vi "MessageBase.getParameters.vi"(8 "error in":errorcluster, 10 "Variant":variant, 11 "MessageBase in":refnum<class "MessageBase.lvclass">) -> (0 "error out":errorcluster, 2 "Variant":variant, 3 "MessageBase out":refnum<class "MessageBase.lvclass">)   [LabVIEW 2020, in "MessageBase.lvclass"]
uses:
  MessageBase.lvclass
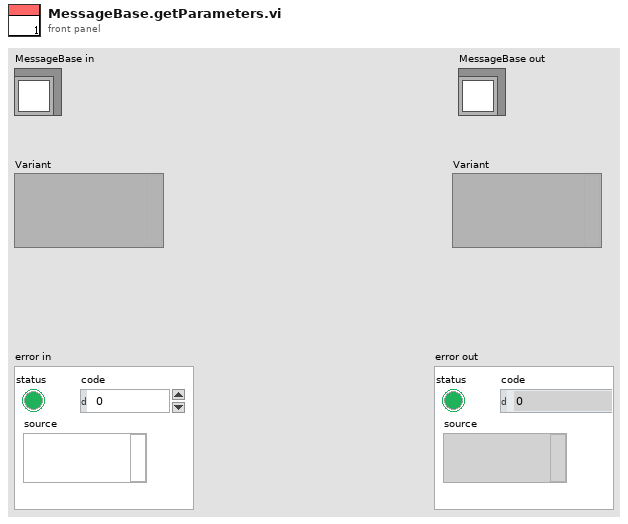
[diagram p1: front panel]
types:
  T1 = typedef "FieldSpec.ctl" = cluster{"Name":string, "Offset":i32, "Length":i32, "FieldType":enum16{"Alphanumeric", "Binary", "BinaryLongPrice", "BinaryShortPrice", "BitField", "PrintableAscii", "Value"}, "FieldValue":variant}
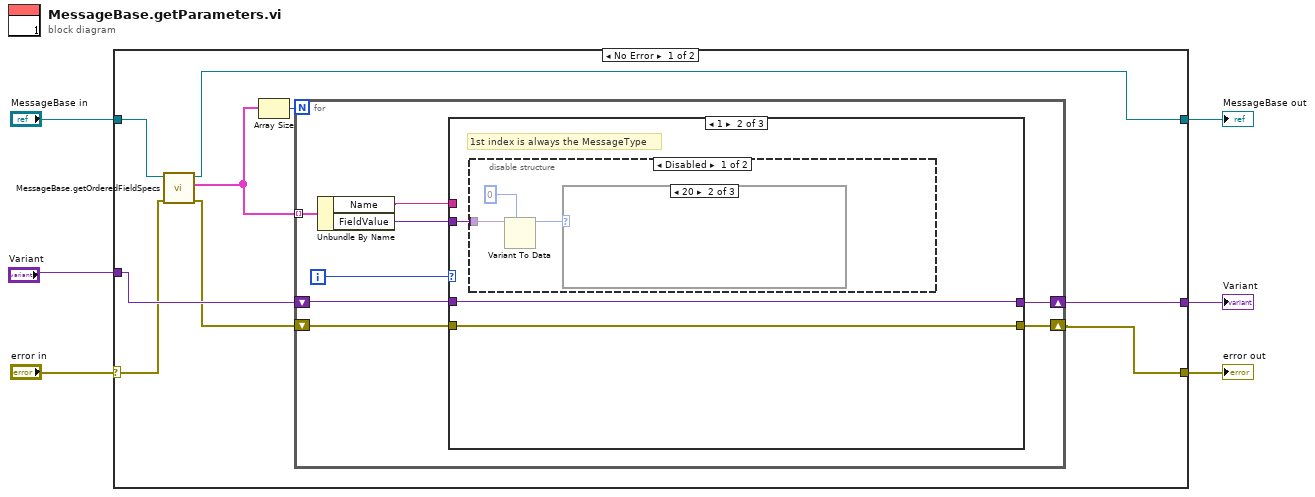
[diagram p0: block diagram]
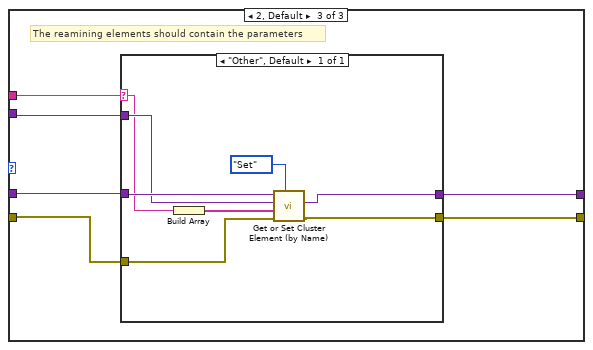
[diagram p6: hidden frame]
diagram:
  n1 = case shown="No Error" "error in" {
    selector: "error in" -> [w10 w47]
    tunnel: [w8 w47] -> w5
    tunnel: [w9 w46] -> w3
    tunnel: "MessageBase in" -> [w14 w46]
    tunnel: "Variant" -> [w12 _]
    tunnel: [w11 _] -> w1
    frame No Error {
      n2 = call-dynamic "MessageBase.getOrderedFieldSpecs.vi"("error in (no error)"=w10, "MessageBase in"=w14) -> ("error out"=w7:errorcluster, "OrderedFieldSpecs"=w13:T1[], "MessageBase out"=w9:refnum<class "MessageBase.lvclass">)  [unwired: 7 in]
      n3 = Array Size(array=w13) -> (size(s)=w15:i32)
      n4 = for {
        N: w15 -> [_]
        tunnel: w13 -> [w23] mode=indexing
        shift-right: [w19] -> w11
        shift-left: w12 -> [w18]
        shift-right: [w17] -> w8
        shift-left: w7 -> [w16]
        i -> [w22]
        n5 = Unbundle By Name(w23) -> ("Name"=w20:string, "FieldValue"=w21:variant)
        n6 = case shown="1" w22 {
          tunnel: w21 -> [_ w28 w36]
          tunnel: w20 -> [_ _ w37]
          tunnel: [w25 w27 w35] -> w19
          tunnel: w18 -> [w25 w27 w34]
          tunnel: [w24 w26 w33] -> w17
          tunnel: w16 -> [w24 w26 w32]
          frame 0 {
            # "0th element is the Message Length"
          }
          frame 1 {
            # "1st index is always the MessageType"
            n7 = disable-structure shown="Disabled" {
              disable-tunnel: w28 -> [w30 _]
              frame Disabled {
                n8 = Variant To Data(type=u8 0, Variant=w30) -> (data=w29:u8)  [unwired: 1 in, 1 out]
                n9 = case shown="20" w29 {
                  frame 0, Default {
                  }
                  frame 32 {
                  }
                  frame 33 {
                  }
                }
              }
              frame Enabled {
              }
            }
          }
          frame 2, Default {
            # "The reamining elements should contain the parameters"
            n10 = case shown="\"Other\", Default" w37 {
              selector: w37 -> [w42]
              tunnel: w34 -> [w45]
              tunnel: w36 -> [w44]
              tunnel: [w41] -> w35
              tunnel: [w39] -> w33
              tunnel: w32 -> [w38]
              frame "Other", Default {
                n11 = Build Array(w42) -> (w43:string[])
                n12 = call <vilib>:"Get or Set Cluster Element (by Name).vi"("Mode"=enum16{"Get", "Set"}."Set", "error in (no error)"=w38, "Name Indices"=w43, "Set"=w44, "Cluster"=w45) -> ("error out"=w39:errorcluster, "Element"=w41:variant)  [unwired: 4 in, 1 out]
              }
            }
          }
        }
      }
    }
    frame Error {
    }
  }
  "error out" <- w5
  "MessageBase out" <- w3
  "Variant" <- w1
